vi "Subvi clock half.vi"() -> (0 "Output":bool)   [LabVIEW 2017]
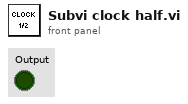
[diagram p1: front panel]
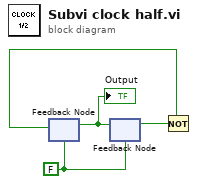
[diagram p0: block diagram]
diagram:
  w1 = FALSE
  n1 = feedback #1(w1) -> (w2:bool)
  "Output" <- w2
  n2 = feedback-in #2(w2) -> ()
  n3 = feedback #2(w1) -> (w4:bool)
  n4 = Not(x=w4) -> (.not. x?=w3:bool)
  n5 = feedback-in #1(w3) -> ()
